vi "Oneof_ConvertClusterToClassTemplate.vi"() -> (0 "OneOfTemplate.lvclass":refnum<class "OneOfTemplate.lvclass">)   [LabVIEW 2019, in "OneOfTemplate.lvclass"]
uses:
  OneOfTemplate.lvclass
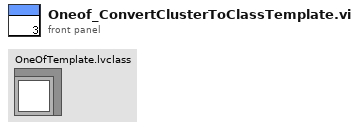
[diagram p1: front panel]
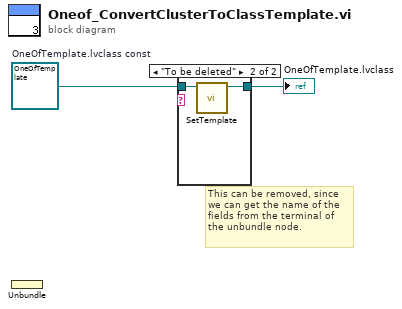
[diagram p0: block diagram]
diagram:
  w2 = refnum<class "OneOfTemplate.lvclass"> refnum  # OneOfTemplate.lvclass const
  # "This can be removed, since\nwe can get the name of the\nfields from the terminal of\nthe unbundle node."
  n1 = Unbundle "Unbundle"() -> ()  [unwired: 1 in, 1 out]
  n2 = case shown="\"To be deleted\"" {
    selector: _ -> [_ _]
    tunnel: w2 -> [w3 w5]
    tunnel: [w3 w4] -> w1
    frame Default {
    }
    frame "To be deleted" {
      n3 = call "SetTemplate.vi"("OneOfTemplate in"=w5) -> ("OneOfTemplate out"=w4:refnum<class "OneOfTemplate.lvclass">)  [unwired: 9 in, 1 out]
    }
  }
  "OneOfTemplate.lvclass" <- w1
